vi "SendChunk.vi"(8 "error in (no error)":errorcluster, 9 "Chunks":string[](array[string]), 10 "index":i32, 11 "WebSocket Server in":refnum<class "WebSocket Server.lvclass">) -> (0 "error out":errorcluster, 1 "Chunk":string, 3 "WebSocket out":refnum<class "WebSocket Server.lvclass">)   [LabVIEW 2018]
uses:
  <vilib>/MediaMongrels Ltd/WebSockets/WebSockets/WebSocket Server/WebSocket Server.lvclass
  <vilib>/addons/Tools/Unicode/UTF8 Tools.lvlib
panel:
  out "Data":u8[](array[numeric]) format="%.0x"
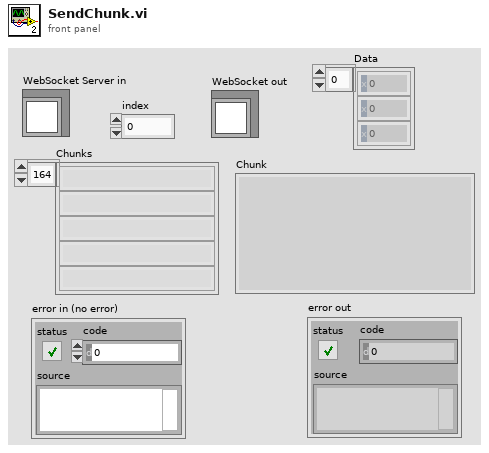
[diagram p1: front panel]
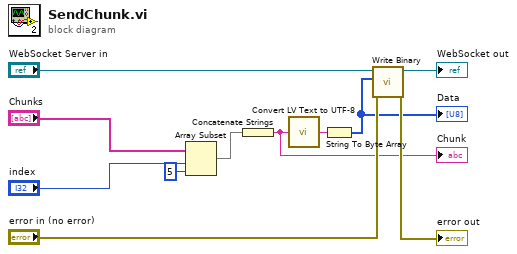
[diagram p0: block diagram]
diagram:
  n1 = Array Subset(array="Chunks", index="index", length=5) -> (w11:string[])
  n2 = Concatenate Strings(w11) -> (w2:string)
  "Chunk" <- w2
  n3 = call <vilib>:"Convert LV Text to UTF-8.vi"("LV Text"=w2) -> ("UTF-8 Text"=w1:string)  [unwired: 13 in, 1 out]
  n4 = String To Byte Array(string=w1) -> (unsigned byte array=w3:u8[])
  "Data" <- w3
  n5 = call-dynamic "Write Binary.vi"("error in (no error)"="error in (no error)", "Binary Data"=w3, "WebSocket in"="WebSocket Server in") -> ("error out"=→"error out":errorcluster, "WebSocket out"=→"WebSocket out":refnum<class "WebSocket Server.lvclass">)  [unwired: 7 in]
